vi "SetFill.vi"(8 "error in (no error)":errorcluster, 10 "Fill":bool, 11 "Polygone in":refnum<class "Polygone.lvclass">) -> (0 "error out":errorcluster, 3 "Polygone out":refnum<class "Polygone.lvclass">)   [LabVIEW 2021, in "Picture2D.lvlib" / "Polygone.lvclass"]
uses:
  Polygone.lvclass
  Polygone.lvclass/Polygone.ctl
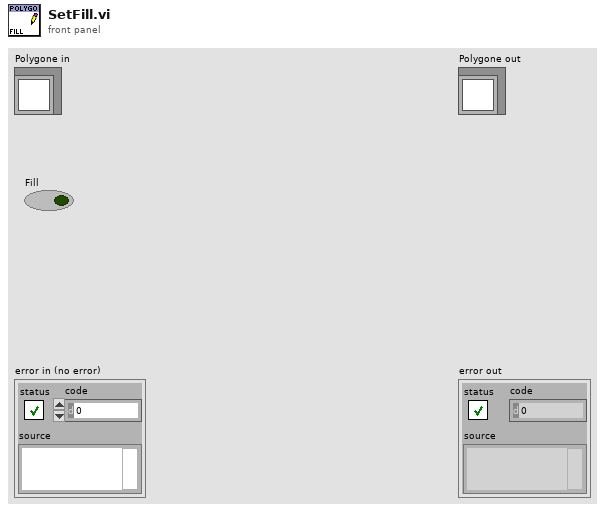
[diagram p1: front panel]
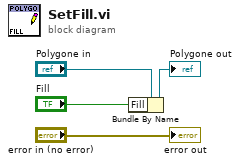
[diagram p0: block diagram]
diagram:
  n1 = Bundle By Name(cluster="Polygone in", "Fill"="Fill") -> (→"Polygone out":refnum<class "Polygone.lvclass">)
  "error out" <- "error in (no error)"
